vi "Interface_Asset_Write Asset.vi"(8 "error in (no error)":errorcluster, 10 "TagBus DVR":refnum<data-value>, 11 "Asset_Interface in":refnum<class "EnergyStorage.lvclass">) -> (0 "error out":errorcluster, 2 "TagBus DVR out":refnum<data-value>, 3 "Asset_Interface out":refnum<class "EnergyStorage.lvclass">)   [LabVIEW 2015, in "EnergyStorage.lvclass"]
uses:
  EnergyStorage.lvclass
  TagBus/TagBus.lvclass
  EnergyStorage_Control.ctl
  EnergyStorage.lvclass/EnergyStorage.ctl
panel:
  in  "Control":T1
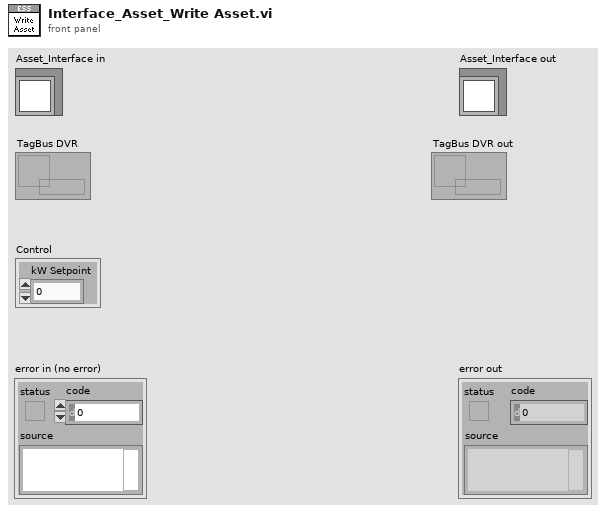
[diagram p1: front panel]
types:
  T1 = typedef "EnergyStorage.lvclass/EnergyStorage_Control.ctl" = cluster{"kW Setpoint":dbl}
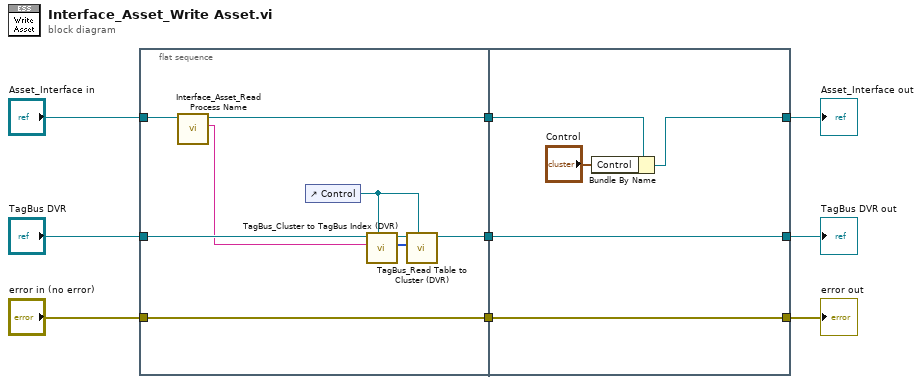
[diagram p0: block diagram]
diagram:
  n1 = flat-sequence {
    tunnel: "TagBus DVR" -> [w18]
    tunnel: [w16] -> w7
    tunnel: "Asset_Interface in" -> [w13]
    tunnel: [w12] -> w5
    tunnel: "error in (no error)" -> [w15]
    tunnel: [w15] -> w2
    tunnel: [w23] -> w8
    tunnel: w7 -> [w23]
    tunnel: w5 -> [w22]
    tunnel: [w21] -> w4
    tunnel: [w20] -> w1
    tunnel: w2 -> [w20]
    frame #0 {
      n2 = call-dynamic "Interface_Asset_Read Process Name.vi"("EnergyStorage in"=w13) -> ("Process Name"=w11:string, "EnergyStorage out"=w12:refnum<class "EnergyStorage.lvclass">)  [unwired: 9 in]
      n3 = control-ref of="Control"() -> (w10:refnum<vi>)
      n4 = call "TagBus_Cluster to TagBus Index (DVR).vi"("Clust Refnum"=w10, "Tag Name Prepend"=w11, "TagBus DVR"=w18) -> ("Index Array"=w14:i32[], "TagBus DVR out"=w17:refnum<data-value>)  [unwired: 7 in]
      n5 = call "TagBus_Read Table to Cluster (DVR).vi"("Clust Refnum"=w10, "Index Array"=w14, "TagBus DVR"=w17) -> ("TagBus DVR out"=w16:refnum<data-value>)  [unwired: 8 in]
    }
    frame #1 {
      n6 = Bundle By Name(cluster=w22, "Control"="Control") -> (w21:refnum<class "EnergyStorage.lvclass">)
    }
  }
  "error out" <- w1
  "Asset_Interface out" <- w4
  "TagBus DVR out" <- w8
